vi "Cache Host Key.vi"(8 "error in (no error)":errorcluster, 11 "Login Info":T1) -> (0 "error out":errorcluster)   [LabVIEW 2023, in "VeriStand Console.lvlib"]
doc: "The first time you connect to a new server, the openSSH library will attempt to connect to the machine, but if the host fingerprint is not cached in the <user>\\.ssh\\known_hosts file, an error will occur. This VI retrieves the key from the SSH host and caches it on the local machine."
uses:
  VeriStand Console.lvlib
  TypeDefs/Login Info.ctl
  <vilib>/Utility/sysdir.llb/System Directory Type.ctl
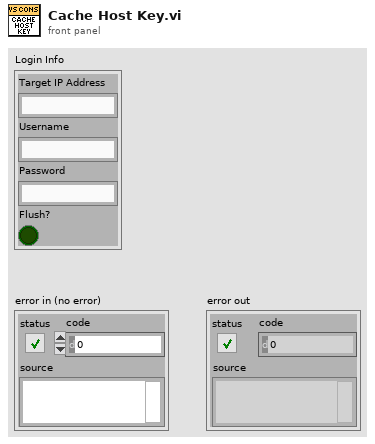
[diagram p1: front panel]
types:
  T1 = typedef "VeriStand Console.lvlib/Login Info.ctl" = cluster{"Target IP Address":string, "Username":string, "Password":string, "Flush?":bool}
  T2 = enum16{"open", "replace", "create", "open or create", "replace or create", "replace or create with confirmation"}
  T3 = typedef "System Directory Type.ctl" = i32
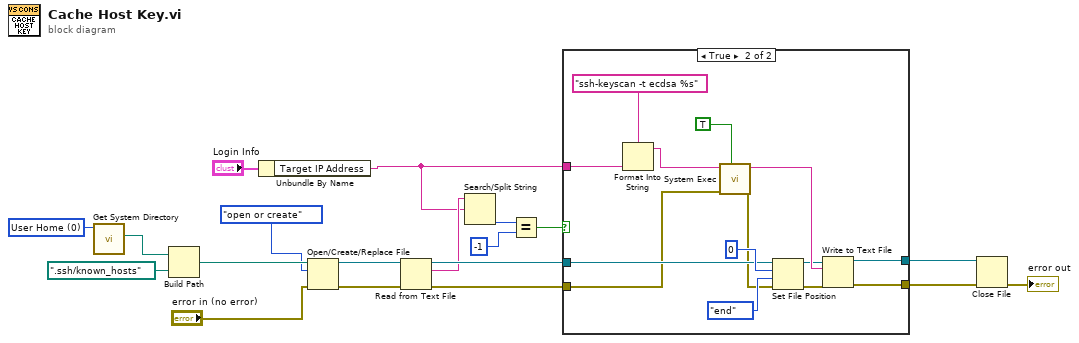
[diagram p0: block diagram]
diagram:
  w18 = T3 0 items=["User Home"=0, "User Desktop"=1, "User Documents"=2, "User Application Data"=3, "User Preferences"=4, "User Temporary"=5, "Public Documents"=6, "Public Application Data"=7, "Public Preferences"=8, "Public Cache"=13, "System Core Libraries"=9, "System Installed Libraries"=10, "Application Files"=11, "Boot Volume Root"=12] ("system directory type")
  n1 = call <vilib>:"Get System Directory.vi"("system directory type"=w18) -> ("system directory"=w17:path)  [unwired: 10 in]
  n2 = Build Path(base path=w17, name or relative path=path ".ssh/known_hosts") -> (appended path=w15:path)
  n3 = Unbundle By Name("Login Info") -> ("Target IP Address"=w6:string)
  n4 = Open/Create/Replace File(file path (use dialog)=w15, error in="error in (no error)", operation (0:open)=T2."open or create") -> (refnum out=w9:refnum<file>, error out=w13:errorcluster)  [unwired: 3 in, 1 out]
  n5 = Read from Text File(file (use dialog)=w9, error in=w13) -> (refnum out=w8:refnum<file>, text=w7:string, error out=w10:errorcluster)  [unwired: 2 in, 1 out]
  n6 = Search/Split String(string=w7, search string/char (-)=w6) -> (offset of match=w5:i32)  [unwired: 1 in, 2 out]
  n7 = Equal?(x=w5, y=-1) -> (x = y?=w3:bool)
  n8 = case shown="True" w3 {
    tunnel: [w20 w32] -> w12
    tunnel: [w21 w31] -> w11
    tunnel: w10 -> [w20 w23]
    tunnel: w8 -> [w21 w25]
    tunnel: w6 -> [_ w24]
    frame False {
      # "Key is already present, don't write to it"
    }
    frame True {
      n9 = Format Into String(format string="ssh-keyscan -t ecdsa %s", w24) -> (resulting string=w34:string)  [unwired: 2 in, 1 out]
      n10 = call <vilib>:"System Exec.vi"("run minimized? (F)"=TRUE, "error in (no error)"=w23, "command line"=w34) -> ("error out"=w22:errorcluster, "standard output"=w30:string)  [unwired: 5 in, 2 out]
      n11 = Set File Position(offset (in bytes) (0)=i64 0, refnum=w25, from (0:start)=enum16{"start", "end", "current"}."end", error in=w22) -> (refnum out=w28:refnum<file>, error out=w29:errorcluster)
      n12 = Write to Text File(file (use dialog)=w28, text=w30, error in=w29) -> (refnum out=w31:refnum<file>, error out=w32:errorcluster)  [unwired: 1 in, 1 out]
    }
  }
  n13 = Close File(refnum=w11, error in=w12) -> (error out=→"error out":errorcluster)  [unwired: 1 out]
